vi "IncStepsNI.vi"(0 "Motion Settings In":T5={"No Motion?"=FALSE, "Motion System"=enum."NI 735x", "Motion Bd ID"=1, "Motion Profile"="SMAC1", "# Axis"=1, "Reverse Z axis?"=TRUE, "SMAC Axis"=0, "scan pair"=enum."y-(x) scan", "RT fps"=6.0, "Steps per mm"=[1000, 1000, 1000, 1000], "Motor Parameters"={"velocity ct/s"=[10000.0, 10000.0, 10000.0, 50000.0], "accel ct/s^2"=[50000.0, 50000.0, 50000.0, 200000.0]}, "One Way Scan"=FALSE, "Reverse One Way Scan"=FALSE, "Global Position (mm)"=[], "Plane"=0, "Distance between\nscan lines (um)"=0.0, "Distance between\nscan planes (um)"=0.0, "number of scan planes"=1, "Total steps in line"=0, "Xtra plane\ndistance  (um)"=100, "Xtra planes "=1, "Add Axis"=FALSE, "overshoot cts"=200, "BKPT Shift"=0, "Scan Start Time (ms)"=0, "ESP VISA"="GPIB::1::INSTR", "3rd Axis"=1, "GL Ref Out"=refnum, "Galil Address"=""} {"3rd Axis" items=["x", "y", "z", "w"]; "Xtra planes" min=1; "Xtra plane\ndistance  (um)" min=0; "Distance between\nscan planes (um)" format="%.2f"; "Distance between\nscan lines (um)" format="%.2f"; "SMAC Axis" items=["None"=0, "Axis 1"=1, "Axis 2"=2, "Axis 3"=3, "Axis 4"=4, "Axis 5"=5, "Axis 6"=6, "Axis 7"=7, "Axis 8"=8, "Vector Space 1"=17, "Vector Space 2"=18, "Vector Space 3"=19, "Vector Space 4"=20]; "Motion Bd ID" min=1 max=32 step=1}, 1 "AlazarCluster":T13, 3 "Avg Num":i32=1, 5 "scans lines":i32=128, 7 "Digitizer Settings":T9={"Digitizer delay (us) "=0.0, "rf points per line"=2048, "lines per plane"=128, "Samp Rate (Hz)"=100000000.0, "Additional dig delay (us)"=0.0, "Voltage Scale"=0.4, "Pre-Looks"=0, "Offset delay (us)"=0.0, "bits A/D"=8, "Avg Num"=1, "DigTimeOut"=5.0, "Rel Dig Delay"=0.0, "Dig Ch"=0, "LeCroyCluster"={"LeCroy Channels"=[TRUE, FALSE, FALSE, FALSE], "LC read pt offset"=0.0, "Sweep Avg"=FALSE}, "Main Digitizer"=enum."NI Digitizer", "Dig Config"=enum."Single channel", "Digitizer ID Cluster"={"Acqiris/Alazar/SP ID"=[], "NI Instr Handles"=[], "LeCroy VISA"="", "GaGe Handle"={"Handle"=0, "Sample size"=0, "Resolution"=0, "Offset"=0, "Channels"=0, "Boards"=0}, "ATS Ref"="ATS9350", "Acqiris Address"=["PCI::INSTR0"], "ADQRef"=refnum, "adq_cu_ptr"=refnum}, "Trigger Settings"={"Trig Source"=1, "Trig Coupling"=0, "Trig Slope"=0, "Level (mV)"=1500.0}, "Bulk Acq"=FALSE, "Bulk Start Indexes"=[], "Data Ref RF"=refnum, "NI ID/Channel"=[], "Total Dig CH"=1, "Xtra Ann Trig delay (us)"=10.0, "Fix Z Delay?"=FALSE, "One Way Transmission?"=FALSE, "Data Ref Log"=refnum} {"Trigger Settings"."Trig Slope" items=["Positive", "Negative"]; "Trigger Settings"."Level (mV)" format="%.2f"; "Trigger Settings"."Trig Coupling" items=["DC 1 MOhm", "AC 1 MOhm", "DC 50 Ohm", "AC 50 Ohm"]; "Trigger Settings"."Trig Source" items=["Chan 1", "External"]; "Rel Dig Delay" format="%.2f"; "DigTimeOut" format="%.2f"; "Avg Num" min=1; "Offset delay (us)" format="%.2f"; "Additional dig delay (us)" format="%.2f"; "Digitizer delay (us)" format="%.2f"}, 9 "Axis":i32=1 min=1 max=4, 11 "File Names":string[](array[string]), 12 "motion error in":errorcluster, 13 "Type of scan":T1, 14 "Reverse ?":bool) -> (15 "Motion error":bool)   [LabVIEW 2022 SP3]
uses:
  Digitizers/-DigitizerRoutines/DigitizerSettings.ctl
  Digitizers/-DigitizerRoutines/Digitizer.ctl
  Digitizers/-DigitizerRoutines/DigConfig.ctl
  Digitizers/-DigitizerRoutines/DigitizerID.ctl
  C:/Windows/System32/ADQAPI_dotNet_helper.dll
  Windows/System32/ADQAPI_dotNet_helper.dll
  MotionParameters.ctl
  MotionSys.ctl
  -MotionRoutines/ScanAxis.ctl
  -MotionRoutines/3rdAxis.ctl
  Annular Array/-AnnularRoutines/AnnularArray.ctl
  Annular Array/-AnnularRoutines/TransGeometry.ctl
  Annular Array/-AnnularRoutines/ArrayGeometry.ctl
  -ScanSystem/Controls/ScanType2.ctl
  Galil/Command Menu.ctl
  <vilib>/Analysis/baseanly.llb/Mean (DBL).vi
  <vilib>/DAQmx/write.llb/DAQmx Write (Digital 1D Bool NChan 1Samp 1Line).vi
  -MotionRoutines/MotionGlobals.vi
  <vilib>/DAQmx/miscellaneous.llb/DAQmx Fill In Error Info.vi
  <instrlib>/Acqiris Dx/Acqiris Dx.lvlib
  <vilib>/Motion/FlexMotion/CustomControls/CustomControls.llb/Program.flx
  <vilib>/Analysis/NI_AALBase.lvlib
  <instrlib>/LeCroy Wave Series/LeCroy Wave Series.lvlib
panel:
  in  "Ann Array Params":T2={"Synth Foc?"=FALSE, "Focal Zones"=41, "Switch T/R"=0, "Trans Geometry (mm)"={"Transducer"=0, "Geo Focus"=12.0, "a (radius)"=3.0, "# of rings"=5, "kerf space "=0.1, "Center Freq"=12.0}, "Sub Ap Excite?"=FALSE, "Full Array Scan?"=FALSE, "Xmt/Rcv"={"XMIT"=[TRUE, TRUE, TRUE, TRUE, TRUE], "RCV"=[TRUE, TRUE, TRUE, TRUE, TRUE]}, "PulseSpacing (us)"=0.0, "Xmit Ring"=0, "XMIT CHS"=0, "RCV CHS"=0, "GPU?"=FALSE, "Save TIFF?"=FALSE, "downfactor"=1, "RCV 1CH"=0} {"RCV 1CH" items=["All", "1", "2", "3", "4", "5"]; "Trans Geometry (mm)"."Transducer" items=["6D 12R 40 MHz"=0, "10D 31R 20 MHz"=1, "10D 23R 20 MHz"=2, "6D 23R 40 MHz"=3, "4.5D 10.7R 40 MHz"=4, "9D 23.5R 20 MHz"=5, "9D 25.8R 20MHz"=6, "Enter"=99]; "Switch T/R" min=1 max=5 step=1}
  out "Intensity Graph":i16[][](graph)
  in  "Acq error in":errorcluster
  # "1-D and 2-D B scan settings"
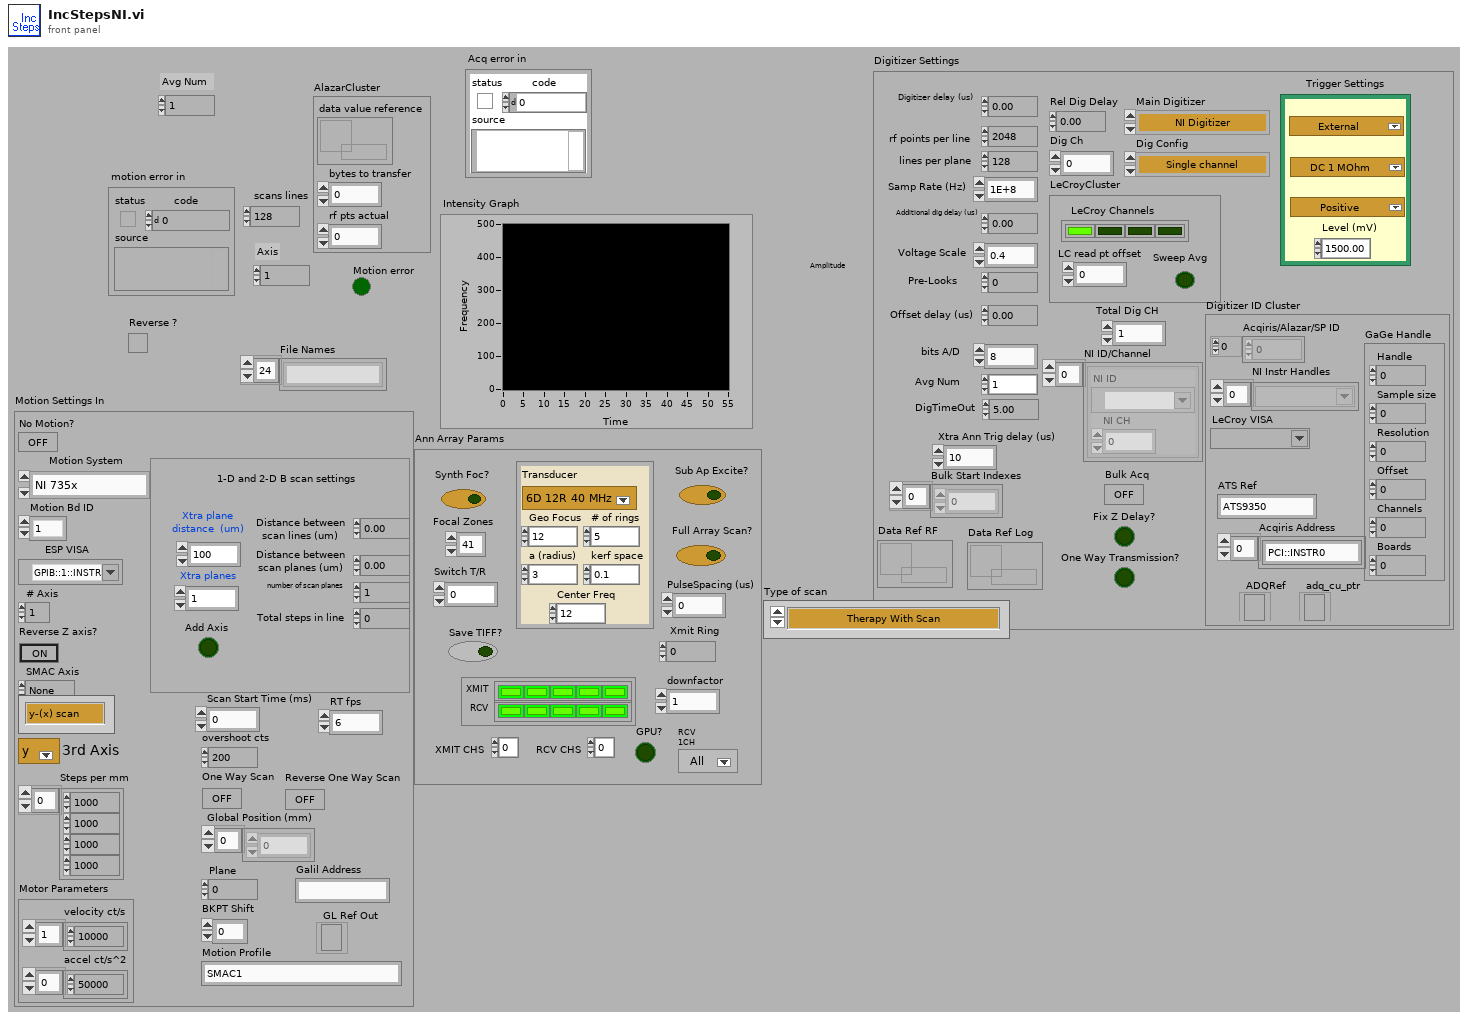
[diagram p1: front panel]
types:
  T1 = typedef "ScanType2.ctl" = enum16{"Therapy With Scan", "M scan", "M Scan With Therapy Burst", "1-D B Scan", "1-D B Scan With Therapy Burst", "2-D B Scan", "2-D B Scan With Therapy Burst", "Rotational Scan", "1-D B-Scan PRF", "2-D B-Scan PRF", "Real-Time Scan", "Contrast Agents", "1-D w/ Real-Time Set Up", "Dual Transducer", "Acoustic Microscopy", "Hydrophone Scanning"}
  T2 = typedef "AnnularArray.ctl" = cluster{"Synth Foc?":bool, "Focal Zones":i16, "Switch T/R":i16, "Trans Geometry (mm)":T3, "Sub Ap Excite?":bool, "Full Array Scan?":bool, "Xmt/Rcv":cluster{"XMIT":bool[], "RCV":bool[]}, "PulseSpacing (us)":sgl, "Xmit Ring":i32, "XMIT CHS":u8, "RCV CHS":u8, "GPU?":bool, "Save TIFF?":bool, "downfactor":i32, "RCV 1CH":u16}
  T3 = typedef "TransGeometry.ctl" = cluster{"Transducer":T4, "Geo Focus":dbl, "a (radius)":dbl, "# of rings":i32, "kerf space ":dbl, "Center Freq":dbl}
  T4 = typedef "ArrayGeometry.ctl" = u16
  T5 = typedef "MotionParameters.ctl" = cluster{"No Motion?":bool, "Motion System":T6, "Motion Bd ID":u8, "Motion Profile":string, "# Axis":i8, "Reverse Z axis?":bool, "SMAC Axis":u16, "scan pair":T7, "RT fps":sgl, "Steps per mm":i32[], "Motor Parameters":cluster{"velocity ct/s":dbl[], "accel ct/s^2":dbl[]}, "One Way Scan":bool, "Reverse One Way Scan":bool, "Global Position (mm)":dbl[], "Plane":i32, "Distance between\nscan lines (um)":sgl, "Distance between\nscan planes (um)":sgl, "number of scan planes":i32, "Total steps in line":i32, "Xtra plane\ndistance  (um)":i32, "Xtra planes ":i32, "Add Axis":bool, "overshoot cts":i32, "BKPT Shift":i32, "Scan Start Time (ms)":u32, "ESP VISA":refnum<visa-resource-name>, "3rd Axis":T8, "GL Ref Out":refnum<k7>, "Galil Address":string}
  T6 = typedef "MotionSys.ctl" = enum16{"MM3000", "NI 735x", "Newport ESP", "No Motion Card", "Galil"}
  T7 = typedef "ScanAxis.ctl" = enum16{"y-(x) scan", "x-(y) scan", "z-(x) scan", "z-(y) scan", "y-(z) scan", "x-(z) scan", "w-(x) scan", "w-(y) scan", "w-(z) scan", "x-(w) scan", "y-(w) scan", "z-(w) scan"}
  T8 = typedef "3rdAxis.ctl" = u16
  T9 = typedef "DigitizerSettings.ctl" = cluster{"Digitizer delay (us) ":dbl, "rf points per line":i32, "lines per plane":i32, "Samp Rate (Hz)":dbl, "Additional dig delay (us)":dbl, "Voltage Scale":dbl, "Pre-Looks":i32, "Offset delay (us)":dbl, "bits A/D":i8, "Avg Num":i32, "DigTimeOut":sgl, "Rel Dig Delay":sgl, "Dig Ch":i32, "LeCroyCluster":cluster{"LeCroy Channels":bool[], "LC read pt offset":dbl, "Sweep Avg":bool}, "Main Digitizer":T10, "Dig Config":T11, "Digitizer ID Cluster":T12, "Trigger Settings":cluster{"Trig Source":u16, "Trig Coupling":u16, "Trig Slope":u16, "Level (mV)":dbl}, "Bulk Acq":bool, "Bulk Start Indexes":i32[], "Data Ref RF":refnum<data-value>, "NI ID/Channel":cluster{"NI ID":refnum<k15>, "NI CH":i32}[], "Total Dig CH":i32, "Xtra Ann Trig delay (us)":dbl, "Fix Z Delay?":bool, "One Way Transmission?":bool, "Data Ref Log":refnum<data-value>}
  T10 = typedef "Digitizer.ctl" = enum16{"Acqiris Digitizer", "NI Digitizer", "LeCroy", "GaGe", "AlazarTech", "No Digitizer", "Teledyne"}
  T11 = typedef "DigConfig.ctl" = enum16{"Single channel", "2 Chans w/ 2 Acqiris", "2 Chans w/ 1 Acqiris", "5-CH Pulser New", "5-CH pulser w/ ann array", "5-pass style ann array", "Empty"}
  T12 = typedef "DigitizerID.ctl" = cluster{"Acqiris/Alazar/SP ID":u32[], "NI Instr Handles":refnum<k15>[], "LeCroy VISA":refnum<visa-resource-name>, "GaGe Handle":cluster{"Handle":u32, "Sample size":u32, "Resolution":i32, "Offset":i32, "Channels":u32, "Boards":u32}, "ATS Ref":string, "Acqiris Address":string[], "ADQRef":refnum<k24>, "adq_cu_ptr":refnum<k24>}
  T13 = cluster{"data value reference":refnum<data-value>, "bytes to transfer":u32, "rf pts actual":u32}
  T14 = enum16{"Absolute Position", "Relative Position", "Velocity", "Relative to Cap Pos", "Modulus Position", "Absolute Contouring", "Relative Contouring"}
  T15 = typedef "Program.flx" = u8
  T16 = typedef "Command Menu.ctl" = enum16{"CommandPassThrough", "Abort Motion", "Define Pos", "Velocity", "Acceleration", "Deceleration", "Position Rel", "Postion Abs", "Begin Move", "After Move", "Home", "KI", "KD", "KP", "IL", "Config I/O", "Set Bit", "Clear Bit", "Motor Off", "Moto On", "Status", "Execute", "Halt Execute", "HX Status", "Tell Velocity", "Check Motion", "BreakPoint", "Tell Position", "Current Code Line", "Tell Switches", "OC Force On", "OC Off", "Pos Soft Limit", "Rev Soft Limit"}
  T17 = typedef "location.ctl" = enum16{"Automatic", "WCM Main", "Hawaii", "Columbia MM3000", "Columbia  NI System", "NYU", "RRI 2", "UHI Allen", "CUMC RT", "Chiba", "Stony Brook", "WCM Microscopy", "WCM Aeoretch", "WCM Optics Lab", "WCM Main 2Axis", "WCM Rotation", "WCM SAM SMAC", "SERI GP"}
  T18 = typedef "Breath_Mode.ctl" = u16
  T19 = cluster{"Reserved":bool, "Axis #1 Move Complete":bool, "Axis #2 Move Complete":bool, "Axis #3 Move Complete":bool, "Axis #4 Move Complete":bool, "Axis #5 Move Complete":bool, "Axis #6 Move Complete":bool, "Axis #7 Move Complete":bool, "Axis #8 Move Complete":bool, "Axis #9 MoveComplete":bool, "Axis #10 Move Complete":bool, "Axis #11 Move Complete":bool, "Axis #12 Move Complete":bool, "Status #13":bool, "Status #14":bool, "Status #15":bool}
  T20 = cluster{"Run/Stop":bool, "Profile Complete":bool, "Motor Off ":bool, "Following Error":bool, "Limit Switch":bool, "Home Switch":bool, "SW Limit Switch":bool, "Watchdog":bool, "Velocity Threshold":bool, "Position Brkpt":bool, "Home Found":bool, "Index Found":bool, "High Speed Capture":bool, "Reverse Direction":bool, "Blend Complete":bool, "Move Complete":bool}
  T21 = cluster{"Handle":u32, "Sample size":u32, "Resolution":i32, "Offset":i32, "Channels":u32, "Boards":u32}
  T22 = cluster{sgl, "Gain [dB]  ":sgl, "Atten (dB)":sgl}[]
  T23 = typedef "SpectrometerType.ctl" = u16
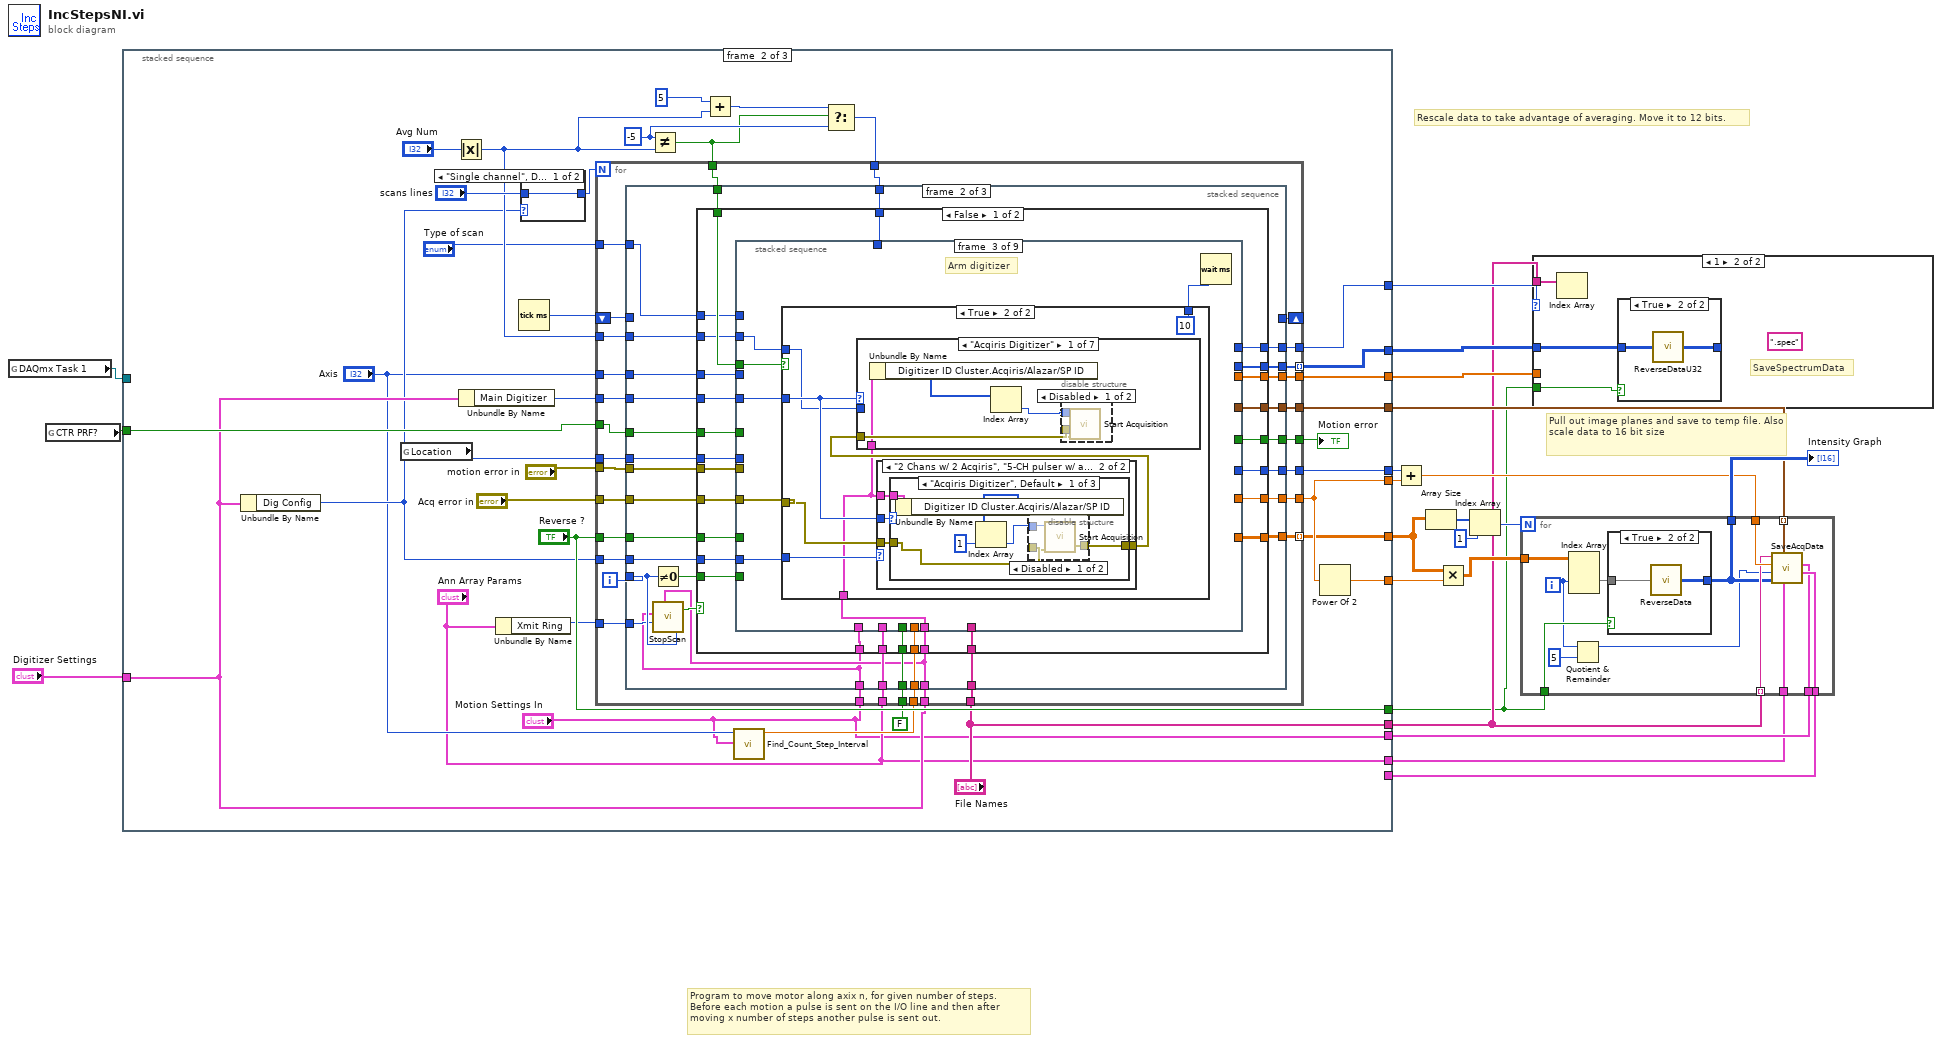
[diagram p0: block diagram]
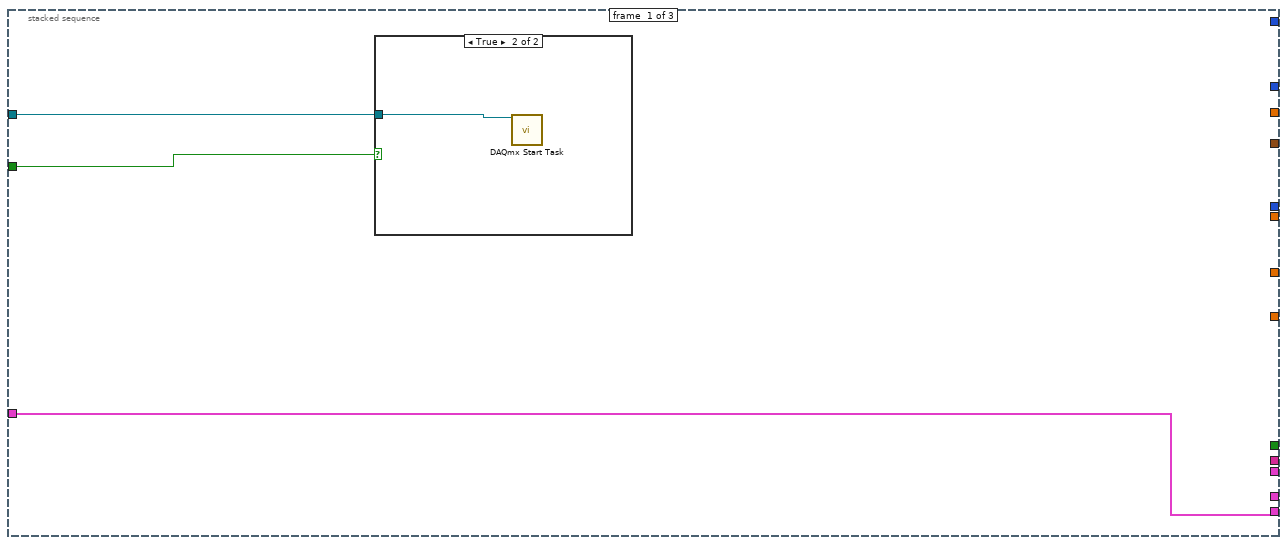
[diagram p4: hidden frame]
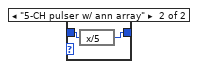
[diagram p6: hidden frame]
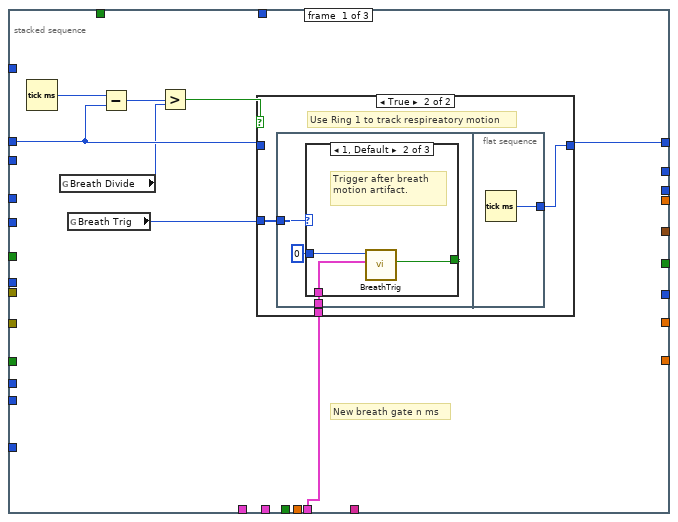
[diagram p7: hidden frame]
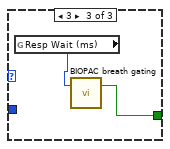
[diagram p10: hidden frame]
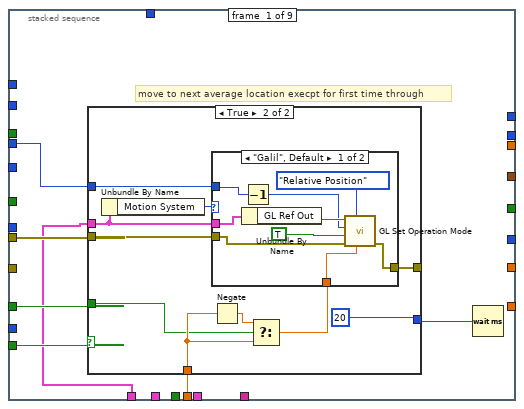
[diagram p11: hidden frame]
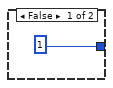
[diagram p12: hidden frame]
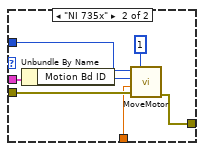
[diagram p13: hidden frame]
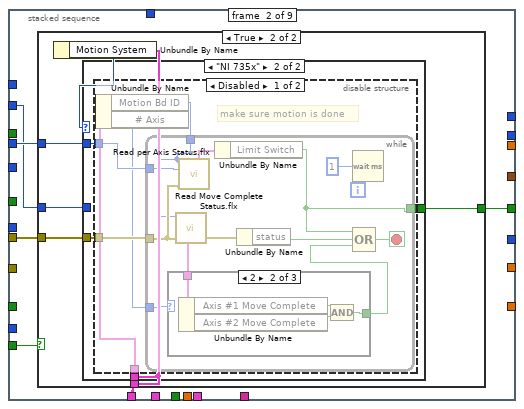
[diagram p14: hidden frame]
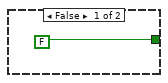
[diagram p15: hidden frame]
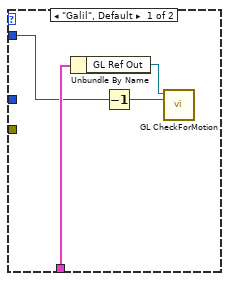
[diagram p16: hidden frame]
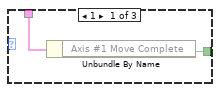
[diagram p17: hidden frame]
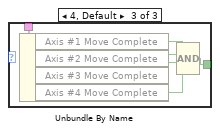
[diagram p18: hidden frame]
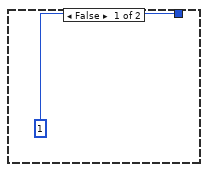
[diagram p20: hidden frame]
diagram:
  # "Pull out image planes and save to temp file. Also scale data to 16 bit size"
  # "Rescale data to take advantage of averaging. Move it to 12 bits."
  # "Program to move motor along axix n, for given number of steps.\nBefore each motion a pulse is sent on the I/O line and then after\nmoving x number of steps another pulse is sent out."
  n1 = global read "MotionGlobals.vi" "DAQmx Task 1"() -> (w10:refnum<k21>)
  n2 = global read "MotionGlobals.vi" "CTR PRF?"() -> (w11:bool)
  n3 = stacked-sequence {
    tunnel: [_ "Reverse ?" _] -> w5
    tunnel: [_ "File Names" _] -> w6
    tunnel: [_ w50 _] -> w18
    tunnel: [_ w49 _] -> w17
    tunnel: [_ w48 _] -> w15
    tunnel: [_ w44 _] -> w14
    tunnel: [_ w43 _] -> w13
    tunnel: w11 -> [w25 w42 w485]
    tunnel: w10 -> [w24 _ w486]
    tunnel: [_ w38 _] -> w8
    tunnel: [_ w37 _] -> w7
    tunnel: [_ w36 _] -> w9
    tunnel: "Digitizer Settings" -> [w23 w34 _]
    tunnel: [w23 _ _] -> w3
    tunnel: [_ "Motion Settings In" _] -> w2
    tunnel: [_ "Ann Array Params" _] -> w1
    frame #0 {
      n4 = case shown="True" w25 {
        tunnel: w24 -> [_ w26]
        frame False {
        }
        frame True {
          n5 = call <vilib>:"DAQmx Start Task.vi"("task/channels in"=w26) -> ()  [unwired: 13 in, 2 out]
        }
      }
    }
    frame #1 {
      w57 = -5
      n6 = Unbundle By Name(w34) -> ("Dig Config"=w32:T11)
      n7 = global read "MotionGlobals.vi" "Location"() -> (w52:T17)
      n8 = Absolute Value(x="Avg Num") -> (abs(x)=w39:i32)
      n9 = Unbundle By Name(w34) -> ("Main Digitizer"=w33:T10)
      n10 = Unbundle By Name("Ann Array Params") -> ("Xmit Ring"=w29:i32)
      n11 = Tick Count (ms)() -> (millisecond timer value=w47:u32)
      n12 = case shown="\"Single channel\", Default" w32 {
        tunnel: "scans lines" -> [w62 w64]
        tunnel: [w62 w63] -> w45
        frame "Single channel", Default {
        }
        frame "5-CH pulser w/ ann array" {
          n13 = expression code="x/5"(w64) -> (w63:i32)
        }
      }
      n14 = Not Equal?(x=w57, y=w39) -> (x != y?=w54:bool)
      n15 = Add(x=5, y=w39) -> (x+y=w55:i32)
      n16 = call "Find_Count_Step_Interval.vi"("Motion Settings In"="Motion Settings In", "Axis"="Axis") -> ("BP Interval"=w35:dbl)  [unwired: 8 in, 1 out]
      n17 = Select(t=w55, s=w54, f=w57) -> (s? t:f=w58:i32)
      n18 = for {
        N: w45 -> [_]
        tunnel: "motion error in" -> [w94]
        tunnel: "Axis" -> [w93]
        tunnel: [w90] -> w60
        tunnel: "Reverse ?" -> [w92]
        tunnel: w58 -> [w91]
        tunnel: "Acq error in" -> [w89]
        tunnel: w32 -> [w88]
        tunnel: [w86] -> w43 mode=indexing
        tunnel: w54 -> [w87]
        tunnel: [w85] -> w49
        tunnel: w39 -> [w84]
        tunnel: w29 -> [w79]
        tunnel: w35 -> [w82]
        tunnel: w33 -> [w81]
        tunnel: w52 -> [w80]
        tunnel: [w78] -> w48
        tunnel: "File Names" -> [w77]
        tunnel: [w76] -> w50
        shift-right: [w74] -> _
        shift-left: w47 -> [w75]
        tunnel: w42 -> [w73]
        tunnel: FALSE -> [w72]
        tunnel: [w71] -> w38 mode=indexing
        tunnel: [w70] -> w37
        tunnel: [w69] -> w36
        tunnel: w34 -> [w68]
        tunnel: "Motion Settings In" -> [w67]
        tunnel: "Ann Array Params" -> [w66]
        tunnel: "Type of scan" -> [w65]
        i -> [w83]
        n19 = stacked-sequence {
          tunnel: w94 -> [_ w145 _]
          tunnel: w93 -> [_ w144 _]
          tunnel: w92 -> [_ w143 _]
          tunnel: w91 -> [_ w142 _]
          tunnel: [_ w141 _] -> w90
          tunnel: w89 -> [_ w140 _]
          tunnel: w88 -> [_ w139 _]
          tunnel: w87 -> [_ w138 _]
          tunnel: [_ w136 _] -> w86
          tunnel: [_ w135 _] -> w85
          tunnel: w84 -> [_ w133 _]
          tunnel: w83 -> [_ w132 _]
          tunnel: w82 -> [_ w131 _]
          tunnel: w81 -> [_ w130 _]
          tunnel: w80 -> [_ w129 _]
          tunnel: w79 -> [_ w128 _]
          tunnel: [_ w127 _] -> w78
          tunnel: w77 -> [_ w126 _]
          tunnel: [_ w125 _] -> w76
          tunnel: w75 -> [w97 _ _]
          tunnel: [w98 _ _] -> w74
          tunnel: w73 -> [_ w124 _]
          tunnel: w72 -> [_ w123 _]
          tunnel: [_ w122 _] -> w71
          tunnel: [_ w121 _] -> w70
          tunnel: [_ w120 _] -> w69
          tunnel: w68 -> [w95 w117 w481]
          tunnel: w67 -> [_ w116 _]
          tunnel: w66 -> [_ w119 _]
          tunnel: w65 -> [_ w118 _]
          frame #0 {
            # "New breath gate n ms"
            n20 = Tick Count (ms)() -> (millisecond timer value=w101:u32)
            n21 = global read "MotionGlobals.vi" "Breath Divide"() -> (w96:i32)
            n22 = global read "MotionGlobals.vi" "Breath Trig"() -> (w102:T18)
            n23 = Subtract(x=w101, y=w97) -> (x-y=w100:u32)
            n24 = Greater?(x=w100, y=w96) -> (0:w99:bool)
            n25 = case shown="True" w99 {
              tunnel: w102 -> [_ w106]
              tunnel: [w103 w105] -> w98
              tunnel: w97 -> [w103 _]
              tunnel: w95 -> [_ w104]
              frame False {
              }
              frame True {
                # "Use Ring 1 to track respireatory motion"
                n26 = flat-sequence {
                  tunnel: w106 -> [w109]
                  tunnel: w104 -> [w107]
                  tunnel: [w115] -> w105
                  frame #0 {
                    n27 = case shown="1, Default" w109 {
                      tunnel: [_ w112 w114] -> _
                      tunnel: 0 -> [_ w111 _]
                      tunnel: w107 -> [_ w110 _]
                      frame 0 {
                      }
                      frame 1, Default {
                        # "Trigger after breath motion artifact."
                        n28 = call "BreathTrig.vi"("Digitizer Settings"=w110, "Xmit Ring"=w111) -> ("BINGO"=w112:bool)  [unwired: 4 in, 5 out]
                      }
                      frame 3 {
                        n29 = global read "MotionGlobals.vi" "Resp Wait (ms)"() -> (w113:u32)
                        n30 = call "BIOPAC breath gating.vi"("Resp Wait (ms)"=w113) -> ("Resp Gate"=w114:bool)  [unwired: 2 in]
                      }
                    }
                  }
                  frame #1 {
                    n31 = Tick Count (ms)() -> (millisecond timer value=w115:u32)
                  }
                }
              }
            }
          }
          frame #1 {
            n32 = Not Equal To 0?(x=w132) -> (x != 0?=w137:bool)
            n33 = call "StopScan.vi"("Motion Settings In"=w116, "Ring"=w128, "Digitizer Settings"=w117, "Line Number"=w132) -> ("Stop Now? Dup"=w134:bool)  [unwired: 2 in]
            n34 = case shown="False" w134 {
              tunnel: w145 -> [w172 _]
              tunnel: w144 -> [w171 _]
              tunnel: w143 -> [w170 _]
              tunnel: w142 -> [w169 _]
              tunnel: [w168 FALSE] -> w141
              tunnel: w140 -> [w167 _]
              tunnel: w139 -> [w166 _]
              tunnel: w138 -> [w165 _]
              tunnel: w137 -> [w164 _]
              tunnel: [w163 dbl[][] [] ("Data")] -> w136
              tunnel: [w162 0] -> w135
              tunnel: w133 -> [w161 _]
              tunnel: w131 -> [w160 _]
              tunnel: w130 -> [w159 _]
              tunnel: w129 -> [w158 _]
              tunnel: [w157 _] -> w127
              tunnel: w126 -> [w156 _]
              tunnel: [w155 _] -> w125
              tunnel: w124 -> [w154 _]
              tunnel: w123 -> [w153 _]
              tunnel: [w152 _] -> w122
              tunnel: [w151 _] -> w121
              tunnel: [w150 _] -> w120
              tunnel: w117 -> [w149 _]
              tunnel: w116 -> [w146 _]
              tunnel: w119 -> [w148 _]
              tunnel: w118 -> [w147 _]
              frame False {
                n35 = stacked-sequence {
                  tunnel: w172 -> [w179 w212 _ w327 _ _ _ w446 _]
                  tunnel: w171 -> [w174 w211 _ _ _ _ _ _ _]
                  tunnel: [_ w210 _ _ _ _ _ _ _] -> w168
                  tunnel: w170 -> [w178 _ _ _ _ w414 _ _ _]
                  tunnel: w169 -> [_ _ _ w323 _ _ _ _ _]
                  tunnel: w167 -> [_ _ w260 _ _ w417 _ _ _]
                  tunnel: w166 -> [_ _ w262 _ w374 _ _ _ w466]
                  tunnel: [_ _ _ _ _ w418 _ _ _] -> w163
                  tunnel: w165 -> [_ _ w264 _ _ w420 _ _ _]
                  tunnel: w164 -> [w177 w209 _ _ _ _ _ _ _]
                  tunnel: [_ _ _ _ _ _ _ _ w464] -> w162
                  tunnel: w161 -> [_ w207 w259 _ w372 w419 _ _ w467]
                  tunnel: w160 -> [w175 _ _ _ _ _ _ _ _]
                  tunnel: w159 -> [_ _ w261 _ w375 _ _ _ _]
                  tunnel: w158 -> [_ _ _ w326 _ _ _ w447 _]
                  tunnel: [_ _ _ _ _ _ _ _ w470] -> w157
                  tunnel: w156 -> [_ _ _ _ _ w416 _ _ _]
                  tunnel: [_ _ _ _ _ w415 _ _ _] -> w155
                  tunnel: w154 -> [_ _ _ w325 _ _ _ _ _]
                  tunnel: w153 -> [_ _ _ w324 _ _ _ _ _]
                  tunnel: [_ _ _ _ _ _ w442 _ _] -> w152
                  tunnel: [_ _ _ _ _ _ w441 _ _] -> w151
                  tunnel: [_ _ _ _ _ _ w440 _ _] -> w150
                  tunnel: w149 -> [_ _ w258 _ w373 w413 _ _ w463]
                  tunnel: w146 -> [w173 w208 _ w322 _ w412 _ w445 _]
                  tunnel: w148 -> [_ _ _ _ _ w411 _ _ _]
                  tunnel: w147 -> [_ _ _ _ _ w410 _ _ _]
                  frame #0 {
                    # "move to next average location execpt for first time through"
                    n36 = case shown="True" w177 {
                      tunnel: w179 -> [_ w190]
                      tunnel: w174 -> [_ w185]
                      tunnel: w178 -> [_ w181]
                      tunnel: [1 20] -> w176
                      tunnel: [_ w187] -> _
                      tunnel: w175 -> [_ w186]
                      tunnel: w173 -> [_ w183]
                      frame False {
                      }
                      frame True {
                        n37 = Unbundle By Name(w183) -> ("Motion System"=w182:T6)
                        n38 = Negate(x=w186) -> (-x=w188:dbl)
                        n39 = Select(t=w188, s=w181, f=w186) -> (s? t:f=w189:dbl)
                        n40 = case shown="\"Galil\", Default" w182 {
                          tunnel: w190 -> [w194 w205]
                          tunnel: w189 -> [w191 w204]
                          tunnel: [w195 w203] -> w187
                          tunnel: w185 -> [w197 w202]
                          tunnel: w183 -> [w199 w201]
                          frame "Galil", Default {
                            n41 = Unbundle By Name(w199) -> ("GL Ref Out"=w198:refnum<k7>)
                            n42 = Decrement(x=w197) -> (x-1=w196:i32)
                            n43 = call "GL Set Operation Mode.vi"("position cts (abs/rel)"=w191, "Position Mode (Absolute)"=T14."Relative Position", "error in (no error)"=w194, "Start Now?"=TRUE, "Axis"=w196, "Galil.IGalil"=w198) -> ("error out"=w195:errorcluster)  [unwired: 3 in, 2 out]
                          }
                          frame "NI 735x" {
                            n44 = Unbundle By Name(w201) -> ("Motion Bd ID"=w200:u8)
                            n45 = call "MoveMotor.vi"("Position Mode (Absolute)"=1, "error in (no error)"=w205, "Target Position (0)"=w204, "Axis or Vector Space"=w202, "Motion Bd ID"=w200) -> ("error out"=w203:errorcluster)  [unwired: 4 in, 2 out]
                          }
                        }
                      }
                    }
                    n46 = Wait (ms)(milliseconds to wait=w176) -> ()  [unwired: 1 out]
                  }
                  frame #1 {
                    n47 = case shown="True" w209 {
                      tunnel: w212 -> [_ w219]
                      tunnel: w211 -> [_ w218]
                      tunnel: [FALSE w217] -> w210
                      tunnel: w208 -> [_ w215]
                      tunnel: w207 -> [_ w216]
                      frame False {
                      }
                      frame True {
                        n48 = Unbundle By Name(w215) -> ("Motion System"=w214:T6)
                        n49 = case shown="\"NI 735x\"" w214 {
                          tunnel: w219 -> [_ w227]
                          tunnel: w218 -> [w220 w226]
                          tunnel: [_ w225] -> w217
                          tunnel: w215 -> [w222 w224]
                          tunnel: w216 -> [_ _]
                          frame "Galil", Default {
                            n50 = Unbundle By Name(w222) -> ("GL Ref Out"=w223:refnum<k7>)
                            n51 = Decrement(x=w220) -> (x-1=w221:i32)
                            n52 = call "GL CheckForMotion.vi"("Axis"=w221, "Refnum in"=w223) -> ()  [unwired: 7 in, 3 out]
                          }
                          frame "NI 735x" {
                            n53 = disable-structure shown="Disabled" {
                              disable-tunnel: w227 -> [w233 _]
                              disable-tunnel: w226 -> [w232 _]
                              disable-tunnel: [w231 _] -> w225
                              disable-tunnel: w224 -> [w230 _]
                              frame Disabled {
                                # "make sure motion is done"
                                n54 = Unbundle By Name(w230) -> ("Motion Bd ID"=w229:u8, "# Axis"=w228:i8)
                                n55 = while {
                                tunnel: w233 -> [w242]
                                tunnel: w232 -> [w241]
                                tunnel: [w237] -> w231
                                tunnel: w228 -> [w235]
                                tunnel: w229 -> [w234]
                                stop <- w236 stop-if-true
                                n56 = call <vilib>:"Read Move Complete Status.flx"("error in (no error)"=w242, "Board ID"=w234) -> ("error out"=w245:errorcluster, "Move Complete Status"=w244:T19)  [unwired: 1 in, 4 out]
                                n57 = case shown="2" w235 {
                                tunnel: w244 -> [w247 w251 w257]
                                tunnel: [w246 w248 w252] -> w238
                                frame 1 {
                                n58 = Unbundle By Name(w247) -> ("Axis #1 Move Complete"=w246:bool)
                                }
                                frame 2 {
                                n59 = Unbundle By Name(w251) -> ("Axis #1 Move Complete"=w249:bool, "Axis #2 Move Complete"=w250:bool)
                                n60 = Compound Arithmetic op=AND(w249, w250) -> (w248:bool)
                                }
                                frame 4, Default {
                                n61 = Unbundle By Name(w257) -> ("Axis #1 Move Complete"=w253:bool, "Axis #2 Move Complete"=w256:bool, "Axis #3 Move Complete"=w255:bool, "Axis #4 Move Complete"=w254:bool)
                                n62 = Compound Arithmetic op=AND(w253, w256, w255, w254) -> (w252:bool)
                                }
                                }
                                n63 = call <vilib>:"Read per Axis Status.flx"("error in (no error)"=w242, "Axis"=w241, "Board ID"=w234) -> ("Per Axis H/W Status"=w240:T20)  [unwired: 6 out]
                                n64 = Unbundle By Name(w240) -> ("Limit Switch"=w237:bool)
                                n65 = Unbundle By Name(w245) -> ("status"=w239:bool)
                                n66 = Wait (ms)(milliseconds to wait=1) -> ()  [unwired: 1 out]
                                n67 = Compound Arithmetic op=OR(w237, w239, w238) -> (w236:bool)
                                }
                              }
                              frame Enabled {
                              }
                            }
                          }
                        }
                      }
                    }
                  }
                  frame #2 {
                    # "Arm digitizer"
                    n68 = case shown="True" w264 {
                      tunnel: [1 10] -> w263
                      tunnel: w262 -> [_ w271]
                      tunnel: w261 -> [_ w270]
                      tunnel: w260 -> [_ w269]
                      tunnel: w259 -> [_ w267]
                      tunnel: w258 -> [_ w266]
                      frame False {
                      }
                      frame True {
                        n69 = case shown="\"2 Chans w/ 2 Acqiris\", \"5-CH pulser w/ ann array\", \"5-pass style ann array\"" w271 {
                          tunnel: w270 -> [_ w304]
                          tunnel: [_ w303] -> w268
                          tunnel: w269 -> [_ w302]
                          tunnel: w266 -> [_ w301]
                          frame "Single channel", Default {
                          }
                          frame "2 Chans w/ 2 Acqiris", "5-CH pulser w/ ann array", "5-pass style ann array" {
                            n70 = case shown="\"Acqiris Digitizer\", Default" w304 {
                              tunnel: [w310 w320 _] -> w303
                              tunnel: w302 -> [w308 w319 _]
                              tunnel: w301 -> [w305 w316 _]
                              frame "Acqiris Digitizer", Default {
                                n71 = Unbundle By Name(w305) -> ("Digitizer ID Cluster.Acqiris/Alazar/SP ID"=w307:u32[])
                                n72 = Index Array(array=w307, index=1) -> (element=w306:u32)
                                n73 = disable-structure shown="Disabled" {
                                disable-tunnel: [w313 _] -> w310
                                disable-tunnel: w308 -> [w312 _]
                                disable-tunnel: w306 -> [w311 _]
                                frame Disabled {
                                n74 = call <instrlib>:"Start Acquisition.vi"("error in (no error)"=w312, "Instrument ID"=w311) -> ("error out"=w313:errorcluster)  [unwired: 2 in, 1 out]
                                }
                                frame Enabled {
                                }
                                }
                              }
                              frame "NI Digitizer" {
                                n75 = Unbundle By Name(w316) -> ("Digitizer ID Cluster.NI Instr Handles"=w315:refnum<k15>[])
                                n76 = Index Array(array=w315, index #1=1 ("index")) -> (element #1=w317:refnum<k15>, element #2=w314:refnum<k15>)  [unwired: 1 in]
                                n77 = call <instrlib>:"niScope Initiate Acquisition.vi"("instrument handle"=w317, "error in"=w319) -> ("error out"=w321:errorcluster)  [unwired: 13 out]
                                n78 = call <instrlib>:"niScope Initiate Acquisition.vi"("instrument handle"=w314, "error in"=w321) -> ("error out"=w320:errorcluster)  [unwired: 13 out]
                              }
                              frame "LeCroy", "No Digitizer" {
                              }
                            }
                          }
                        }
                        n79 = case shown="\"Acqiris Digitizer\"" w270 {
                          tunnel: w268 -> [w276 w282 w287 _ w290 _ w297]
                          tunnel: w267 -> [_ _ w286 _ _ _ _]
                          tunnel: w266 -> [w273 w279 w285 w289 w291 _ w300]
                          frame "Acqiris Digitizer" {
                            n80 = Unbundle By Name(w273) -> ("Digitizer ID Cluster.Acqiris/Alazar/SP ID"=w275:u32[])
                            n81 = Index Array(array=w275) -> (element=w274:u32)  [unwired: 1 in]
                            n82 = disable-structure shown="Disabled" {
                              disable-tunnel: w276 -> [w278 _]
                              disable-tunnel: w274 -> [w277 _]
                              frame Disabled {
                                n83 = call <instrlib>:"Start Acquisition.vi"("error in (no error)"=w278, "Instrument ID"=w277) -> ()  [unwired: 2 in, 2 out]
                              }
                              frame Enabled {
                              }
                            }
                          }
                          frame "NI Digitizer", Default {
                            n84 = Unbundle By Name(w279) -> ("Digitizer ID Cluster.NI Instr Handles"=w281:refnum<k15>[])
                            n85 = Index Array(array=w281) -> (element=w280:refnum<k15>)  [unwired: 1 in]
                            n86 = call <instrlib>:"niScope Initiate Acquisition.vi"("instrument handle"=w280, "error in"=w282) -> ()  [unwired: 14 out]
                          }
                          frame "LeCroy" {
                            n87 = Unbundle By Name(w285) -> ("LeCroyCluster.Sweep Avg"=w283:bool, "Digitizer ID Cluster.LeCroy VISA"=w284:refnum<visa-resource-name>)
                            n88 = call "LeCroyAVG_Arm.vi"("EXT AVG"=w283, "error in"=w287, "Avg Num"=w286, "LeCroy"=w284) -> ()  [unwired: 6 in, 2 out]
                          }
                          frame "GaGe" {
                            n89 = Unbundle By Name(w289) -> ("Digitizer ID Cluster.GaGe Handle"=w288:T21)
                            n90 = call "CsTool-CaptureFill.vi"("Handle Cluster"=w288) -> ()  [unwired: 1 out]
                          }
                          frame "AlazarTech" {
                            n91 = Unbundle By Name(w291) -> ("Digitizer ID Cluster.Acqiris/Alazar/SP ID"=w293:u32[])
                            n92 = Index Array(array=w293) -> (element=w292:u32)  [unwired: 1 in]
                            n93 = call "AlazarStartCapture.vi"("Handle"=w292, "error in (no error)"=w290) -> ()  [unwired: 3 out]
                          }
                          frame "No Digitizer" {
                          }
                          frame "Teledyne" {
                            n94 = Unbundle By Name(w300) -> ("Digitizer ID Cluster.ADQRef"=w299:refnum<k24>, "Digitizer ID Cluster.adq_cu_ptr"=w294:refnum<k24>, "Digitizer ID Cluster.GaGe Handle.Boards"=w295:u32)
                            n95 = call "SPADQ_DisarmArmTrigger.vi"("error in (no error)"=w297, "adq_num"=w295, "adq_cu_ptr in"=w294, "ADQAPI Ref"=w299) -> ("error out"=w296:errorcluster, "ADQAPI Ref (out)"=w298:refnum<k24>)  [unwired: 6 in]
                            n96 = call "SPADQ_ArmTrigger.vi"("error in (no error)"=w296, "adq_num"=w295, "adq_cu_ptr in"=w294, "ADQAPI Ref"=w298) -> ()  [unwired: 6 in, 2 out]
                          }
                        }
                      }
                    }
                    n97 = Wait (ms)(milliseconds to wait=w263) -> ()  [unwired: 1 out]
                  }
                  frame #3 {
                    # "turn on prf"
                    n98 = case shown="\"Hawaii\", \"SERI GP\"" w326 {
                      tunnel: w327 -> [_ w338]
                      tunnel: w323 -> [_ w337]
                      tunnel: w325 -> [w331 _]
                      tunnel: w324 -> [_ w336]
                      tunnel: w322 -> [w329 w335]
                      frame "WCM Main", Default {
                        n99 = case shown="False" w331 {
                          tunnel: [w332 w333] -> w330
                          frame False {
                            w332 = u16 0 items=["Function Gen Input", "Motion Trig", "Internal RT Motion Trig", "Internal CTR 1 Output"] ("Trig Source")
                          }
                          frame True {
                            w333 = u16 3 items=["Function Gen Input", "Motion Trig", "Internal RT Motion Trig", "Internal CTR 1 Output"] ("Trig Source")
                          }
                        }
                        n100 = Unbundle By Name(w329) -> ("GL Ref Out"=w328:refnum<k7>)
                        n101 = call "RouteTrigSource.vi"("Galil.IGalil"=w328, "Trig Source"=w330) -> ()  [unwired: 9 in, 1 out]
                      }
                      frame "Hawaii", "SERI GP" {
                        n102 = Unbundle By Name(w335) -> ("Motion System"=w334:T6)
                        n103 = case shown="\"Galil\"" w334 {
                          tunnel: w338 -> [_ w342 w361]
                          tunnel: w337 -> [_ w339 w360]
                          tunnel: w336 -> [_ w341 w359]
                          tunnel: w335 -> [_ w340 w358]
                          frame "MM3000", Default {
                          }
                          frame "NI 735x" {
                            n104 = disable-structure shown="Disabled" {
                              disable-tunnel: w342 -> [w347 _]
                              disable-tunnel: w339 -> [w346 _]
                              disable-tunnel: w341 -> [w345 _]
                              disable-tunnel: w340 -> [w344 _]
                              frame Disabled {
                                n105 = Unbundle By Name(w344) -> ("Motion Bd ID"=w343:u8)
                                n106 = case shown="False" w345 {
                                tunnel: w343 -> [w350 w353]
                                tunnel: w347 -> [w349 w352]
                                tunnel: w346 -> [_ w351]
                                frame False {
                                n107 = call <vilib>:"Run Program.flx"("error in (no error)"=w349, "Program (1)"=T15 3, "Board ID"=w350) -> ()  [unwired: 3 in, 3 out]
                                }
                                frame True {
                                n108 = for {
                                N: w351 -> [_]
                                tunnel: w353 -> [w356]
                                tunnel: w352 -> [w355]
                                n109 = call "ForceBreakPt.vi"("error in"=w355, "Bd ID in"=w356) -> ()  [unwired: 2 out]
                                n110 = Wait (ms)(milliseconds to wait=3) -> ()  [unwired: 1 out]
                                }
                                }
                                }
                              }
                              frame Enabled {
                              }
                            }
                          }
                          frame "Galil" {
                            n111 = Unbundle By Name(w358) -> ("GL Ref Out"=w357:refnum<k7>)
                            n112 = case shown="True" w359 {
                              tunnel: w357 -> [w363 w368]
                              tunnel: w361 -> [w364 w367]
                              tunnel: w360 -> [_ w366]
                              frame False {
                                n113 = call "GL Command Set.vi"("Command"=Command_Menu."Execute", "Text Input"="#PRF", "error in (no error)"=w364, "Galil.IGalil"=w363) -> ()  [unwired: 3 in, 5 out]
                              }
                              frame True {
                                n114 = for {
                                N: w366 -> [_]
                                tunnel: w368 -> [w370]
                                tunnel: w367 -> [w369]
                                n115 = call "GL_ForceBreakPt.vi"("error in"=w369, "GL Ref Out"=w370) -> ()  [unwired: 2 out]
                                n116 = Wait (ms)(milliseconds to wait=3) -> ()  [unwired: 1 out]
                                }
                              }
                            }
                          }
                        }
                      }
                    }
                  }
                  frame #4 {
                    # "Wait for segs if using Acqiris"
                    n117 = case shown="\"Acqiris Digitizer\", Default" w375 {
                      tunnel: w372 -> [w382 _ w397 _ _]
                      tunnel: [w380 _ _ _ _] -> _
                      tunnel: w374 -> [w381 _ _ _ _]
                      tunnel: w373 -> [w379 _ w396 w399 w409]
                      frame "Acqiris Digitizer", Default {
                        n118 = Unbundle By Name(w379) -> ("Digitizer ID Cluster.Acqiris/Alazar/SP ID"=w378:u32[])
                        n119 = Index Array(array=w378) -> (element #1=w377:u32, element #2=w376:u32)  [unwired: 2 in]
                        n120 = disable-structure shown="Disabled" {
                          disable-tunnel: w382 -> [w388 _]
                          disable-tunnel: w381 -> [w387 _]
                          disable-tunnel: [w385 _] -> w380
                          disable-tunnel: w377 -> [w384 _]
                          disable-tunnel: w376 -> [w383 _]
                          frame Disabled {
                            n121 = call "WaitForSegs.vi"("Acqiris ID"=w384, "lines per plane"=w388) -> ("error out"=w386:errorcluster)  [unwired: 2 in, 3 out]
                            n122 = case shown="\"2 Chans w/ 2 Acqiris\", \"5-pass style ann array\"" w387 {
                              tunnel: w383 -> [_ w393]
                              tunnel: w388 -> [_ w391]
                              tunnel: w386 -> [_ w390]
                              tunnel: [_ w389] -> w385
                              frame "Single channel", Default {
                              }
                              frame "2 Chans w/ 2 Acqiris", "5-pass style ann array" {
                                n123 = call "WaitForSegs.vi"("Acqiris ID"=w393, "lines per plane"=w391, "error in"=w390, "Timeout"=500) -> ("error out"=w389:errorcluster)  [unwired: 3 out]
                              }
                            }
                          }
                          frame Enabled {
                          }
                        }
                      }
                      frame "NI Digitizer", "No Digitizer" {
                      }
                      frame "LeCroy" {
                        n124 = Unbundle By Name(w396) -> ("LeCroyCluster.Sweep Avg"=w394:bool, "Digitizer ID Cluster.LeCroy VISA"=w395:refnum<visa-resource-name>)
                        n125 = call "LeCroyAVG_Wait.vi"("EXT AVG"=w394, "Avg Num"=w397, "LeCroy"=w395) -> ()  [unwired: 7 in, 2 out]
                      }
                      frame "GaGe" {
                        n126 = Unbundle By Name(w399) -> ("Digitizer ID Cluster.GaGe Handle"=w398:T21)
                        n127 = while {
                          tunnel: w398 -> [w400]
                          stop <- w401 stop-if-true
                          n128 = call "CsTool-QueryStatusAll.vi"("Handle Cluster"=w400) -> ("Status"=w402:i32)
                          n129 = Less Or Equal To 0?(x=w402) -> (x <= 0?=w401:bool)
                        }
                      }
                      frame "Teledyne" {
                        n130 = Unbundle By Name(w409) -> ("Digitizer ID Cluster.ADQRef"=w408:refnum<k24>, "Digitizer ID Cluster.adq_cu_ptr"=w407:refnum<k24>, "Digitizer ID Cluster.GaGe Handle.Boards"=w406:u32, "DigTimeOut"=w405:sgl)
                        n131 = Multiply(x=w405, y=sgl 1000.0) -> (x*y=w404:sgl)
                        n132 = call "SPADQ_AcquisitionStatus.vi"("WaitTime (ms)"=w404, "adq_num"=w406, "adq_cu_ptr in"=w407, "ADQAPI Ref"=w408) -> ()  [unwired: 4 in, 4 out]
                      }
                    }
                  }
                  frame #5 {
                    n133 = case shown="True" w420 {
                      tunnel: w419 -> [_ w433]
                      tunnel: [_ w431] -> w418
                      tunnel: w417 -> [_ w430]
                      tunnel: w416 -> [_ w429]
                      tunnel: [_ w428] -> _
                      tunnel: [_ w427] -> w415
                      tunnel: w414 -> [_ w426]
                      tunnel: w413 -> [_ w424]
                      tunnel: w412 -> [_ w423]
                      tunnel: w411 -> [_ w422]
                      tunnel: w410 -> [_ w421]
                      frame False {
                      }
                      frame True {
                        # "File names just for program flow"
                        n134 = call "GetData.vi"("AlazarCluster"="AlazarCluster", "Digitizer Settings"=w424, "Ann Array Params"=w422, "Motion Settings"=w423, "All files"=w429, "error in"=w430, "lines per plane mod"=w433, "Type of scan"=w421, "save?"=FALSE, "Reverse ?"=w426) -> ("Gain Array"=w427:T22, "Raw data out"=w432:i16[][][], "error out"=w428:errorcluster)  [unwired: 7 in]
                        n135 = for {
                          tunnel: w432 -> [w437] mode=indexing
                          tunnel: [w435] -> w431 mode=indexing
                          n136 = Transpose 2D Array(2D array=w437) -> (transposed array=w436:i16[][])
                          n137 = for {
                            tunnel: w436 -> [w439] mode=indexing
                            tunnel: [w438] -> w435 mode=indexing
                            n138 = call-poly <vilib>:"Mean.vi"("X"=w439) -> ("mean"=w438:dbl)  [unwired: 1 out]
                          }
                        }
                      }
                    }
                  }
                  frame #6 {
                    # "Get Spectrum"
                    n139 = global read "MotionGlobals.vi" "Main Spectrometer"() -> (w440:T23)
                    n140 = case shown="1" w440 {
                      tunnel: [_ u32[] [] ("Spectrum")] -> w442
                      tunnel: [_ dbl[] [] ("Wavelengths")] -> w441
                      frame 0, Default {
                      }
                      frame 1 {
                        # "OceanGetSpectrumLV"
                      }
                    }
                  }
                  frame #7 {
                    # "turn off prf"
                    n141 = case shown="\"Hawaii\"" w447 {
                      tunnel: w446 -> [_ w452]
                      tunnel: w445 -> [_ w451]
                      frame "WCM Main", Default {
                        n142 = call-poly <vilib>:"DAQmx Write.vi"("task/channels in"=refnum<k21> "DIO-L2 L3", "data"=bool[] [TRUE, FALSE]) -> ()  [unwired: 11 in, 3 out]
                      }
                      frame "Hawaii" {
                        n143 = Unbundle By Name(w451) -> ("Motion System"=w450:T6)
                        n144 = case shown="\"NI 735x\"" w450 {
                          tunnel: w452 -> [_ w454 _]
                          tunnel: w451 -> [_ w453 w462]
                          frame "MM3000", Default {
                          }
                          frame "NI 735x" {
                            n145 = disable-structure shown="Disabled" {
                              disable-tunnel: w454 -> [w457 _]
                              disable-tunnel: w453 -> [w456 _]
                              frame Disabled {
                                n146 = Unbundle By Name(w456) -> ("Motion Bd ID"=w455:u8)
                                n147 = call <vilib>:"Stop Program.flx"("error in (no error)"=w457, "Program (1)"=T15 3, "Board ID"=w455) -> ()  [unwired: 3 in, 3 out]
                              }
                              frame Enabled {
                              }
                            }
                          }
                          frame "Galil" {
                            n148 = Unbundle By Name(w462) -> ("GL Ref Out"=w461:refnum<k7>)
                            n149 = call "GL Command Set.vi"("Command"=Command_Menu."Halt Execute", "Value"=-1, "Galil.IGalil"=w461) -> ()  [unwired: 4 in, 5 out]
                          }
                        }
                      }
                    }
                  }
                  frame #8 {
                    # "choose bits for final save format"
                    n150 = case shown="\"5-CH pulser w/ ann array\"" w466 {
                      tunnel: w467 -> [w475 w476]
                      tunnel: [w474 w476] -> w465
                      frame "5-CH pulser w/ ann array" {
                        n151 = expression code="x/5"(w475) -> (w474:i32)
                      }
                      frame "2 Chans w/ 2 Acqiris", Default {
                      }
                    }
                    n152 = Logarithm Base 2(1:w465) -> (0:w473:dbl)
                    n153 = Unbundle By Name(w463) -> ("bits A/D"=w464:i8)
                    n154 = Round Toward +Infinity(x=w473) -> (ceil(x): smallest int >= x=w472:dbl)
                    n155 = Subtract(x=16, y=w464) -> (x-y=w468:i32)
                    n156 = In Range and Coerce(upper limit=w468, x=w472, lower limit=0.0) -> (coerced(x)=w470:dbl)  [unwired: 1 out]
                  }
                }
              }
              frame True {
              }
            }
          }
          frame #2 {
            n157 = Unbundle By Name(w481) -> ("LeCroyCluster.Sweep Avg"=w480:bool)
            n158 = case shown="True" w480 {
              tunnel: w481 -> [_ w483]
              frame False {
              }
              frame True {
                n159 = Unbundle By Name(w483) -> ("Digitizer ID Cluster.LeCroy VISA"=w482:refnum<visa-resource-name>)
                n160 = call <instrlib>:"Write.vi"("Write Buffer"="VBS 'app.acquisition.C1.AverageSweeps=1'", "VISA resource name"=w482) -> ()  [unwired: 7 in, 3 out]
              }
            }
          }
        }
      }
      "Motion error" <- w60
      n161 = Power Of 2(x=w48) -> (2^x=w44:dbl)
    }
    frame #2 {
      n162 = case shown="True" w485 {
        tunnel: w486 -> [_ w487]
        frame False {
        }
        frame True {
          n163 = call <vilib>:"DAQmx Stop Task.vi"("task/channels in"=w487) -> ()  [unwired: 13 in, 2 out]
        }
      }
    }
  }
  n164 = Add(x=w17, y=w15) -> (x+y=w16:dbl)
  n165 = Array Size(array=w13) -> (size(s)=w22:i32[])
  n166 = Multiply(x=w13, y=w14) -> (x*y=w12:dbl[][][])
  n167 = Index Array(array=w22, index=1) -> (element=w20:i32)
  n168 = for {
    N: w20 -> [_]
    tunnel: w12 -> [w500]
    tunnel: w5 -> [w499]
    tunnel: w16 -> [w498]
    tunnel: w6 -> [w496] mode=indexing
    tunnel: [w495] -> w19
    tunnel: w18 -> [w494] mode=indexing
    tunnel: w3 -> [w493]
    tunnel: w2 -> [w492]
    tunnel: w1 -> [w488]
    i -> [w491]
    n169 = Index Array(array=w500, index (dim 1)=w491) -> (element=w497:dbl[][])  [unwired: 2 in]
    n170 = Quotient & Remainder(x=w491, y=5) -> (x-y*floor(x/y)=w489:i32)  [unwired: 1 out]
    n171 = case shown="True" w499 {
      tunnel: w497 -> [w502 w504]
      tunnel: [w501 w503] -> w495
      frame False {
        n172 = To Word Integer(number=w502) -> (16bit integer=w501:i16[][])
      }
      frame True {
        n173 = call "ReverseData.vi"("Array in"=w504) -> ("Array out"=w503:i16[][])
      }
    }
    n174 = call "SaveAcqData.vi"("Digitizer Settings"=w493, "Motion Settings"=w492, "Ann Array Params"=w488, "Votage scaling"=w494, "Array"=w495, "Pulser Channel"=w489, "Dig Word Size"=w498, "File Name"=w496) -> ()  [unwired: 3 in]
  }
  "Intensity Graph" <- w19
  n175 = case shown="1" w9 {
    tunnel: w8 -> [_ w506]
    tunnel: w7 -> [_ _]
    tunnel: w6 -> [_ w507]
    tunnel: w5 -> [_ w505]
    frame 0, Default {
    }
    frame 1 {
      (unwired) ".spec" ("Ext")
      # "SaveSpectrumData"
      n176 = Index Array(array=w507) -> ()  [unwired: 1 in, 1 out]
      n177 = case shown="True" w505 {
        tunnel: w506 -> [w508 w509]
        tunnel: [w508 w510] -> _
        frame False {
        }
        frame True {
          n178 = call "ReverseDataU32.vi"("Array in"=w509) -> ("Array out"=w510:u32[][])
        }
      }
    }
  }
